vi "SV 5-1-3 Synchronization Pulse Waveform.vi"(6 "sampling info":cluster{"Fs":dbl, "#s":dbl}={"Fs"=51200.0, "#s"=5120.0} {"Fs" format="%.2p"}, 8 "error in (no error)":errorcluster, 10 "pulse duration (s)":dbl=0.03 format="%_3p", 11 "amplitude":dbl=1.0 format="%.2f") -> (0 "error out":errorcluster, 3 "synchronization pulse":waveform(dbl))   [LabVIEW 2017, in "SoundVib_Generation.lvlib"]
doc: "This VI generates a synchronization pulse waveform that has proven effective for measuring delays in electroacoustic systems. Prepend this signal to an audio test signal to help measure absolute time delay and relative time delays between channels. Append this signal to a test signal to measure time delays and clock drift. When using the output synchronization pulse from this VI as the <b>reference signal</b> input in SV Measure Delay (Equal Polarity) VI, select 'Cross correlation' for the <b>method</b>."
uses:
  <vilib>/addons/_NISVFA/_Generation/SoundVib_Generation.lvlib
  <vilib>/Analysis/4window.llb/Hanning Window (DBL).vi
  <vilib>/Analysis/4window.llb/AllCosWindow (DBL).vi
  <vilib>/Analysis/NI_AALPro.lvlib
  <vilib>/Analysis/NI_AALBase.lvlib
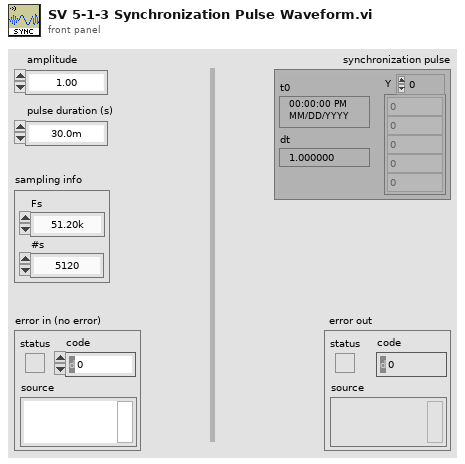
[diagram p1: front panel]
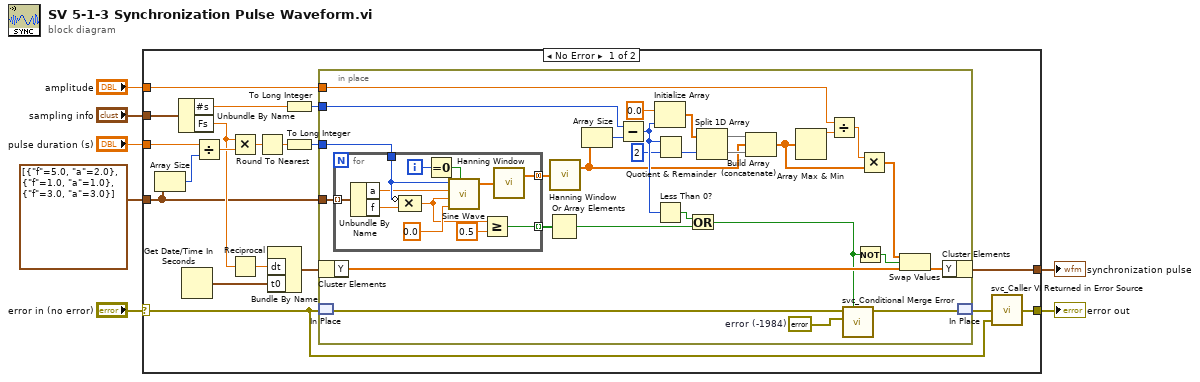
[diagram p0: block diagram]
diagram:
  n1 = case shown="No Error" "error in (no error)" {
    selector: "error in (no error)" -> [w13 w67]
    tunnel: "pulse duration (s)" -> [w26 _]
    tunnel: "sampling info" -> [w24 _]
    tunnel: cluster{"f":dbl, "a":dbl}[] [{"f"=5.0, "a"=2.0}, {"f"=1.0, "a"=1.0}, {"f"=3.0, "a"=3.0}] -> [w8 _]
    tunnel: "amplitude" -> [w19 _]
    tunnel: [w14 _] -> w3
    tunnel: [w11 w67] -> w1
    frame No Error {
      n2 = Array Size(array=w8) -> (size(s)=w25:i32)
      n3 = Unbundle By Name(w24) -> ("#s"=w21:dbl, "Fs"=w16:dbl)
      n4 = Get Date/Time In Seconds() -> (seconds since 1Jan1904=w18:timestamp)
      n5 = Divide(x=w26, y=w25) -> (x/y=w23:dbl)
      n6 = Multiply(x=w16, y=w23) -> (x*y=w22:dbl)
      n7 = Reciprocal(x=w16) -> (1/x=w17:dbl)
      n8 = Round To Nearest(number=w22) -> (nearest integer value=w10:dbl)
      n9 = Bundle By Name("dt"=w17, "t0"=w18) -> (w15:waveform(dbl))  [unwired: 1 out]
      n10 = To Long Integer(number=w21) -> (32bit integer=w20:i32)
      n11 = To Long Integer(number=w10) -> (32bit integer=w9:i32)
      n12 = in-place {
        in-place-border: w8 -> [w53]
        in-place-border: w20 -> [w52]
        in-place-border: w19 -> [w48]
        in-place-border: w9 -> [w36]
        w37 = errorcluster {"status"=TRUE, "code"=-1984, "source"="<append>\nVerify that sample rate, Fs, is more than twice the highest frequency component in the pulse, and verify that the pulse duration is completely generated (#s/Fs >= pulse duration). "}  # error (-1984)
        n13 = in-place-cluster #1(w15) -> ("Y"=w45:dbl[])
        n14 = in-place-match #2(w13) -> (w39:errorcluster)
        n15 = for {
          tunnel: w36 -> [w61]
          tunnel: [w65] -> w54 mode=concatenating
          tunnel: w53 -> [w64] mode=indexing
          tunnel: [w55] -> w42 mode=indexing
          i -> [w59]
          n16 = Unbundle By Name(w64) -> ("a"=w60:dbl, "f"=w63:dbl)
          n17 = Compound Arithmetic op=MULTIPLY(invert w61, w63) -> (w57:dbl)
          n18 = Equal To 0?(x=w59) -> (x = 0?=w58:bool)
          n19 = call <vilib>:"Sine Wave.vi"("samples"=w61, "amplitude"=w60, "frequency"=w57, "phase in"=0.0, "reset phase"=w58) -> ("sine wave"=w62:dbl[])  [unwired: 2 out]
          n20 = Greater Or Equal?(x=w57, y=0.5) -> (x >= y?=w55:bool)
          n21 = call-poly <vilib>:"Hanning Window.vi"("X"=w62) -> ("Windowed X"=w65:dbl[])  [unwired: 1 out]
        }
        n22 = Or Array Elements(Boolean array=w42) -> (logical OR=w40:bool)
        n23 = call-poly <vilib>:"Hanning Window.vi"("X"=w54) -> ("Windowed X"=w27:dbl[])  [unwired: 1 out]
        n24 = Array Size(array=w27) -> (size(s)=w51:i32)
        n25 = Subtract(x=w52, y=w51) -> (x-y=w33:i32)
        n26 = Initialize Array(0.0 ("element"), w33) -> (w31:dbl[])
        n27 = Less Than 0?(x=w33) -> (x < 0?=w41:bool)
        n28 = Quotient & Remainder(x=w33, y=2) -> (floor(x/y)=w30:i32)  [unwired: 1 out]
        n29 = Or(x=w41, y=w40) -> (x .or. y?=w35:bool)
        n30 = Split 1D Array(array=w31, index=w30) -> (first subarray=w28:dbl[], second subarray=w29:dbl[])
        n31 = Build Array (concatenate)(w28, w27, w29) -> (w46:dbl[])
        n32 = Array Max & Min(array=w46) -> (max value=w49:dbl)  [unwired: 3 out]
        n33 = Divide(x=w48, y=w49) -> (x/y=w47:dbl)
        n34 = call <vilib>:"svc_Conditional Merge Error.vi"("merge"=w35, "new error"=w37, "error in (no error)"=w39) -> ("error out"=w38:errorcluster)  [unwired: 8 in]
        n35 = Not(x=w35) -> (.not. x?=w34:bool)
        n36 = Multiply(x=w47, y=w46) -> (x*y=w43:dbl[])
        n37 = Swap Values(12:w43, 13:w34, 14:w45) -> (3:w44:dbl[])  [unwired: 1 out]
        n38 = in-place-cluster #1("Y"=w44) -> (w14:waveform(dbl))
        n39 = in-place-match #2(w38) -> (w12:errorcluster)
      }
      n40 = call <vilib>:"svc_Caller VI Returned in Error Source.vi"("warning input to caller"=w13, "error in (no error)"=w12) -> ("error out"=w11:errorcluster)  [unwired: 3 in]
    }
    frame Error {
    }
  }
  "error out" <- w1
  "synchronization pulse" <- w3
